vi "SVT Limit Testing (XY) (scalar limits).vi"(8 "error in (no error)":errorcluster, 9 "lower limit":dbl=-inf format="%.2f", 10 "upper limit":dbl=inf format="%.2f", 11 "signal in":cluster{"X":dbl[], "Y":dbl[]} {"X" format="%.2f"; "Y" format="%.2f"}) -> (0 "error out":errorcluster, 1 "output values":cluster{"frequencies":dbl[], "spectrum":dbl[]}[](graph), 2 "test results":bool[](array[boolean]), 3 "test passed?":bool)   [LabVIEW 2017]
doc: "Performs limit testing on waveforms, spectra, XY data, identified peaks, or scalar measurements. You can wire <B>output values</B> to a graph to view the limits, signal, and failures. You can use this polymorphic VI to perform limit testing of a waveform, a waveform with scalar limits, a spectrum, a spectrum with scalar limits, XY data, XY data with scalar limits, peaks, peaks with scalar limits, or a scalar value. The data type you wire to the <B>signal in</B> input determines the polymorphic instance to use."
uses:
  <vilib>/addons/Sound and Vibration/svt_Limit Test/SoundVib_LimitTest.lvlib
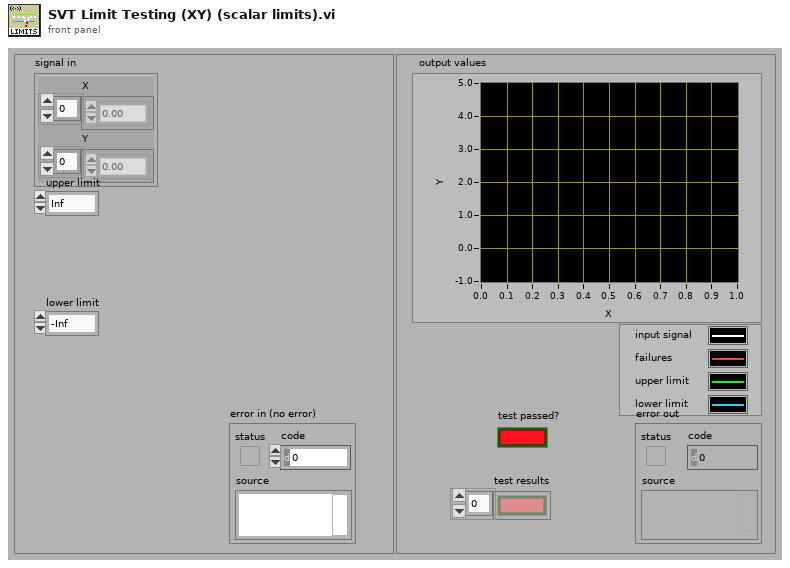
[diagram p1: front panel]
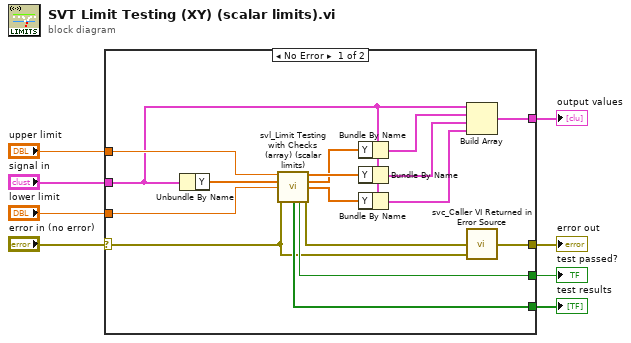
[diagram p0: block diagram]
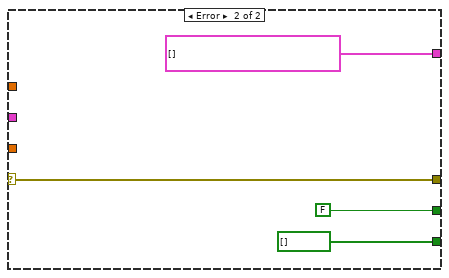
[diagram p2: hidden frame]
diagram:
  n1 = case shown="No Error" "error in (no error)" {
    selector: "error in (no error)" -> [w9 w28]
    tunnel: [w24 w28] -> w7
    tunnel: [w19 cluster{"frequencies":dbl[], "spectrum":dbl[]}[] []] -> w6
    tunnel: [w16 bool[] [] ("Array Constant")] -> w5
    tunnel: [w17 FALSE] -> w4
    tunnel: "signal in" -> [w20 _]
    tunnel: "lower limit" -> [w21 _]
    tunnel: "upper limit" -> [w22 _]
    frame No Error {
      n2 = Unbundle By Name(w20) -> ("Y"=w23:dbl[])
      n3 = call <vilib>:"svl_Limit Testing with Checks (array) (scalar limits).vi"("upper limit"=w22, "input array"=w23, "lower limit"=w21, "error in (no error)"=w9) -> ("upper limit array"=w15:dbl[], "failure array"=w13:dbl[], "lower limit array"=w14:dbl[], "test results"=w16:bool[], "test passed"=w17:bool, "error out"=w18:errorcluster)  [unwired: 6 in]
      n4 = Bundle By Name(cluster=w20, "Y"=w13) -> (w12:cluster{"X":dbl[], "Y":dbl[]})
      n5 = Bundle By Name(cluster=w20, "Y"=w15) -> (w11:cluster{"X":dbl[], "Y":dbl[]})
      n6 = Bundle By Name(cluster=w20, "Y"=w14) -> (w10:cluster{"X":dbl[], "Y":dbl[]})
      n7 = Build Array(w20, w12, w11, w10) -> (w19:cluster{"X":dbl[], "Y":dbl[]}[])
      n8 = call <vilib>:"svc_Caller VI Returned in Error Source.vi"("warning input to caller"=w9, "error in (no error)"=w18) -> ("error out"=w24:errorcluster)  [unwired: 3 in]
    }
    frame Error {
    }
  }
  "error out" <- w7
  "output values" <- w6
  "test passed?" <- w4
  "test results" <- w5
